vi "configuration UI.vi"() -> ()   [LabVIEW 2013, in "file io module editor node.lvclass"]
uses:
  file io module editor node.lvclass
  <vilib>/NI/DCAF UI Toolkit/Controls/Remove.ctl
  <vilib>/NI/DCAF UI Toolkit/Controls/Add.ctl
  <vilib>/NI/Configuration Framework/Node/NodeRef.ctl
  <vilib>/NI/Configuration Framework/Node/NISE_CEF_Node.lvclass
  <vilib>/NI/AMC/Message Queue.ctl
  <vilib>/NI/AMC/Message.ctl
  <vilib>/NI/Tools/Keyed Array/KeyedArray.ctl
  <vilib>/NI/Configuration Framework/Node/UserEventRef.ctl
  <vilib>/NI/Configuration Framework/Controls/EventCluster.ctl
  <vilib>/NI/Configuration Framework/Node/StopEvent.ctl
  <vilib>/NI/Configuration Framework/Node/RefreshUIEvent.ctl
  <vilib>/NI/Configuration Framework/Node/CacheState.ctl
  <vilib>/NI/Configuration Framework/Node/NodeChangeEvent.ctl
  <vilib>/NI/Tag Bus/tag/Data Type.ctl
  <vilib>/NI/Tag Bus Data Framework/control module/editor node/channel action event.ctl
  <vilib>/NI/Tag Bus Data Framework/control module/editor node/dialog output action.ctl
  <vilib>/NI/Tag Bus Module Framework/channel/TBM channel.lvclass
  <vilib>/NI/Tag Bus/tag/tag descriptor.lvclass
  access.ctl
  <vilib>/NI/DCAF Table API/Table Manager/object ref.ctl
  <vilib>/NI/Tag Bus Data Framework/Configuration Editor/Classes/Engine Parent/Engine Parent Editor Node.lvclass
  <vilib>/NI/Tag Bus Data Framework/Configuration Editor/Classes/Module editor node/module editor node.lvclass
  <vilib>/NI/DCAF Table API/Table Manager/references.ctl
  <vilib>/NI/DCAF Table API/Listbox/Multi Column Listbox.lvclass
  <vilib>/Utility/miscctls.llb/LVPositionTypeDef.ctl
  <vilib>/NI/DCAF Table API/Listbox/Multi Column Listbox.lvclass/Multi Column Listbox.ctl
  <vilib>/NI/DCAF Table API/Table Manager/Table Manager.lvclass/Table Manager.ctl
  <vilib>/NI/DCAF Table API/Listbox/Write Listbox.vi
  <vilib>/NI/DCAF Table API/Table Manager/Write Top VI.vi
  <vilib>/NI/Tag Bus Data Framework/control module/editor node/control module editor.lvclass
  <vilib>/NI/DCAF Table API/Table Manager/Table Manager.lvclass
  <vilib>/NI/Tools/Keyed Array/Tools_KeyedArray.lvlib
  <vilib>/NI/AMC/AMC.lvlib
  <vilib>/NI/Configuration Framework/NISE_CEF_TreeControl.lvlib
  <vilib>/NI/DCAF UI Toolkit/Controls/DCAF UI Elements.lvlib
panel:
  in  "data type":T1
  in  "access":T2
  in  "Top Level Tab Control":enum32{"<Main Page>"}(tab)
  in  "tag list box":i32(listbox)=1
  in  "remove tag":T3
  in  "Add tag":T4
  in  "user event out":refnum<user-event>
  in  "node change":T5
  in  "cache state":T6
  in  "refresh UI":T7
  in  "stop event":T8
  in  "user event":T9
  in  "main queue":T10
  in  "node ref":T11
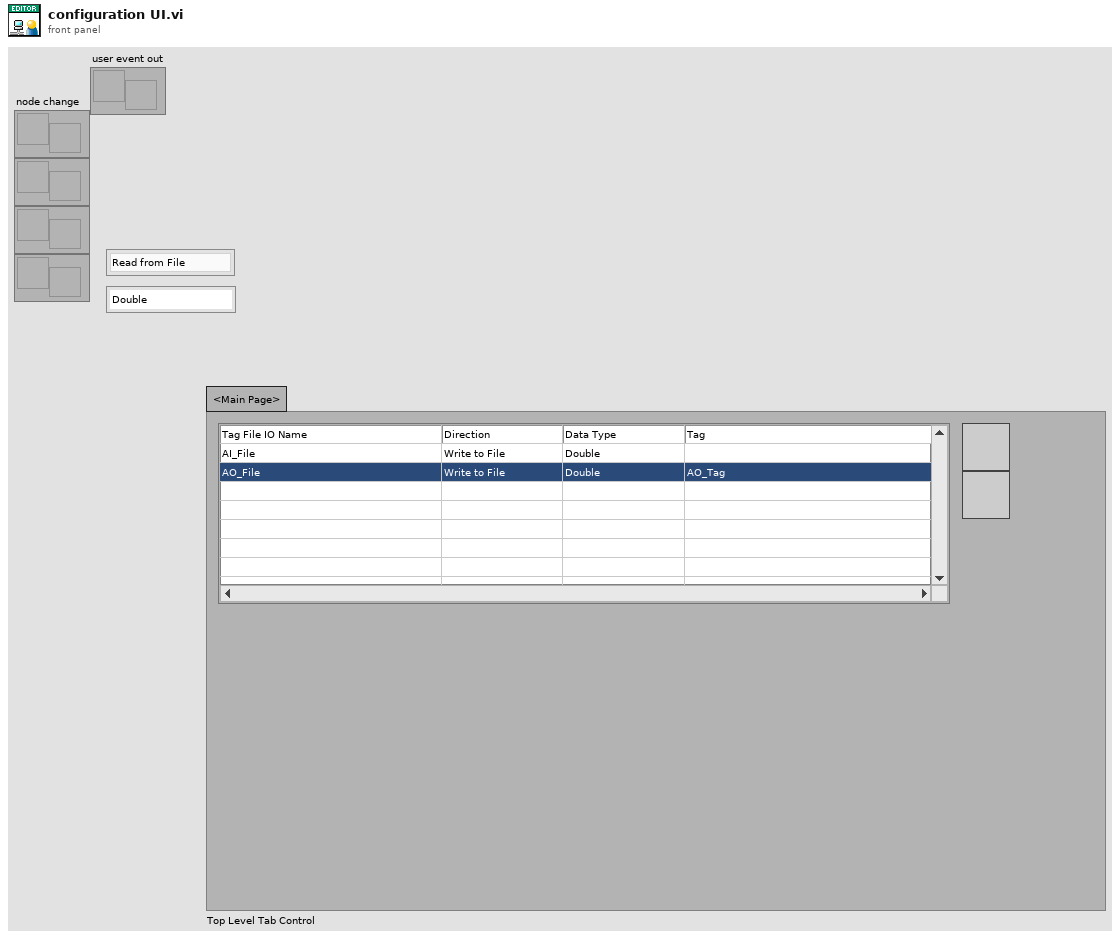
[diagram p1: front panel]
types:
  T1 = typedef "tag bus.lvlib/tag descriptor.lvclass/Data Type.ctl" = enum16{"Double", "Single", "I64", "I32", "I16", "I8", "U64", "U32", "U16", "U8", "Boolean", "String", "Array of Double", "Array of Single", "Array of I64", "Array of I32", "Array of I16", "Array of I8", "Array of U64", "Array of U32", "Array of U16", "Array of U8", "Array of Boolean", "Array of String"}
  T2 = typedef "file io module editor node.lvclass/access.ctl" = enum16{"Read from File", "Write to File"}
  T3 = typedef "DCAF UI Elements.lvlib/Remove.ctl" = bool
  T4 = typedef "DCAF UI Elements.lvlib/Add.ctl" = bool
  T5 = typedef "NISE_CEF_Node.lvclass/NodeChangeEvent.ctl" = refnum<user-event>
  T6 = typedef "NISE_CEF_Node.lvclass/CacheState.ctl" = refnum<user-event>
  T7 = typedef "NISE_CEF_Node.lvclass/RefreshUIEvent.ctl" = refnum<user-event>
  T8 = typedef "NISE_CEF_Node.lvclass/StopEvent.ctl" = refnum<user-event>
  T9 = typedef "NISE_CEF_Node.lvclass/UserEventRef.ctl" = refnum<user-event>
  T10 = typedef "AMC.lvlib/Message Queue.ctl" = refnum<queue>
  T11 = typedef "NISE_CEF_Node.lvclass/NodeRef.ctl" = refnum<data-value>
  T12 = typedef "LVPositionTypeDef.ctl" = cluster{"Left":i32, "Top":i32}
  T13 = typedef "Table Manager.lvlib/Table Manager.lvclass/references.ctl" = cluster{"stop event":T8, "refresh UI":T7, "cache state":T6, "node change":T5, "user event out":refnum<user-event>, "main queue":T10, "user event":T9}
  T14 = typedef "Table Manager.lvlib/Table Manager.lvclass/object ref.ctl" = cluster{"engine":refnum<data-value>, "Node Ref":refnum<data-value>}
  T15 = typedef "Table Manager.lvlib/Column.lvclass/Column Descriptor.ctl" = cluster{"name":string, "caption":string, "Column Type":T16, "Params":string, "AutoSizeMode":i32, "FillWeight":sgl, "MinWidth":u32, "tooltip":string, "Enum Reference":refnum<vi>, "Channel suffix":string, "Read Only":bool, "Call Back VI":T17, "DT Dependency":i32, "name dependency":i32, "data type":T1}
  T16 = typedef "Table Manager.lvlib/Column.lvclass/Column Type.ctl" = enum16{"String", "Mapping", "Channel Name", "Tag", "Enum", "Data Type", "Numeric"}
  T17 = typedef "Table Manager.lvlib/Table Manager.lvclass/Call Back Ref Type Def.ctl" = refnum<vi>
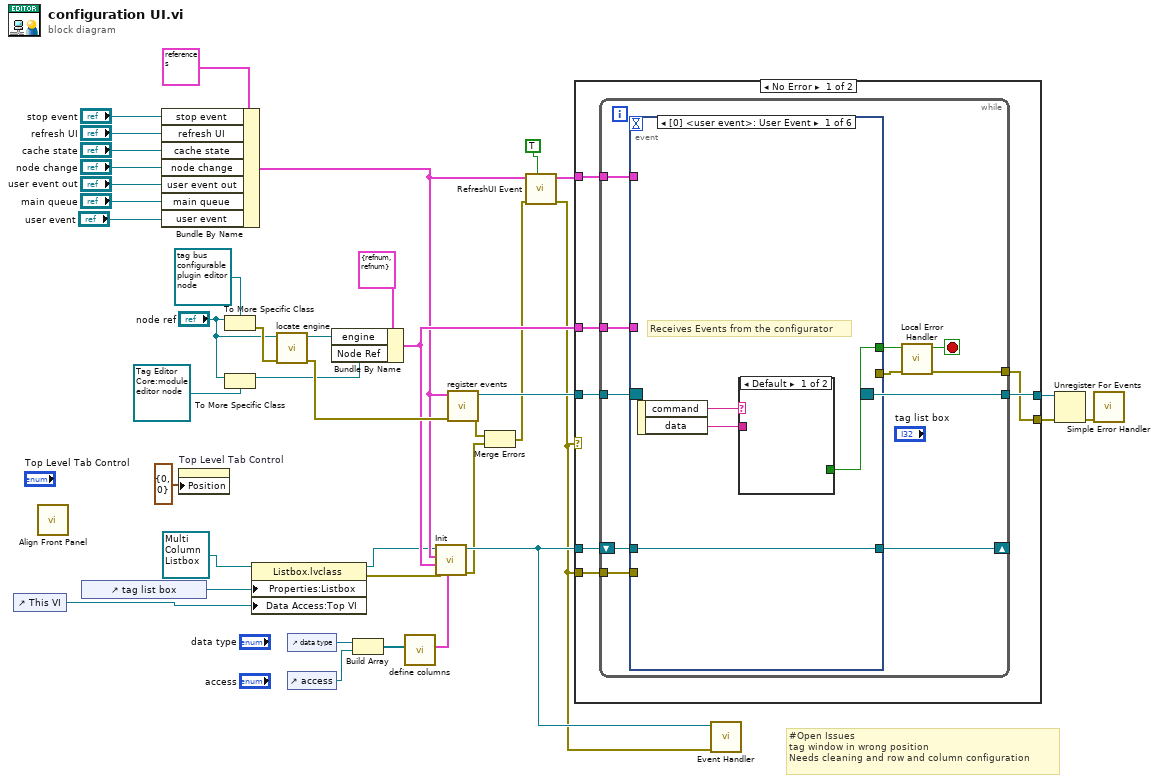
[diagram p0: block diagram]
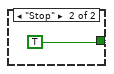
[diagram p2: hidden frame]
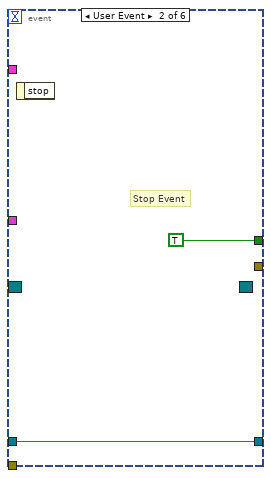
[diagram p3: hidden frame]
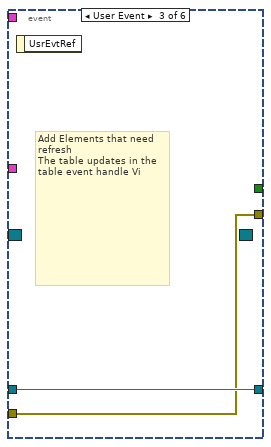
[diagram p4: hidden frame]
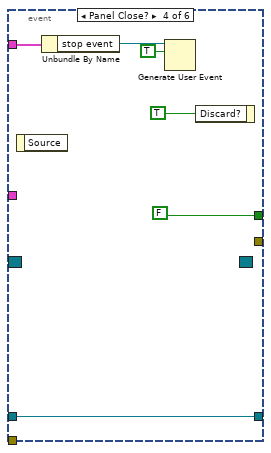
[diagram p5: hidden frame]
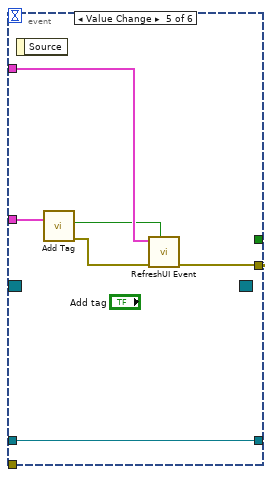
[diagram p6: hidden frame]
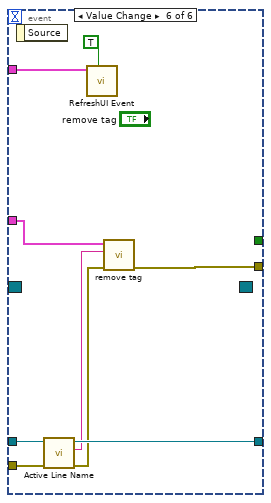
[diagram p7: hidden frame]
diagram:
  # "#Open Issues \ntag window in wrong position\nNeeds cleaning and row and column configuration"
  n1 = control-ref of="This VI"() -> (w15:refnum<vi>)
  n2 = call <vilib>:"Align Front Panel.vi"() -> ()  [unwired: 10 in, 2 out]
  n3 = control-ref of="tag list box"() -> (w16:refnum<vi>)
  n4 = Bundle By Name(cluster=T13 {"stop event"=refnum, "refresh UI"=refnum, "cache state"=refnum, "node change"=refnum, "user event out"=refnum, "main queue"=refnum, "user event"=refnum} ("References"), "stop event"="stop event", "refresh UI"="refresh UI", "cache state"="cache state", "node change"="node change", "user event out"="user event out", "main queue"="main queue", "user event"="user event") -> (w13:T13)
  n5 = property on="Top Level Tab Control" class="TabCtl (strict)"("Position"=T12 {"Left"=0, "Top"=0}) -> ()  [unwired: 2 in, 2 out]
  n6 = To More Specific Class(target class=refnum<data-value> refnum ("data value reference"), reference="node ref") -> (error out=w24:errorcluster)  [unwired: 1 in, 1 out]
  n7 = To More Specific Class(target class=refnum<data-value> refnum ("data value reference"), reference="node ref") -> (specific class reference=w6:refnum<data-value>)  [unwired: 1 in, 1 out]
  n8 = property class="Listbox.lvclass"(reference=refnum<class "Multi Column Listbox.lvclass"> refnum ("Table Manager.lvlib:Multi Column Listbox.lvclass"), "Properties:Listbox"=w16, "Data Access:Top VI"=w15) -> (reference out=w5:refnum<class "Multi Column Listbox.lvclass">, error out=w20:errorcluster)  [unwired: 1 in]
  n9 = call <vilib>:"locate engine.vi"("error in"=w24, "component"="node ref") -> ("error out"=w21:errorcluster, "engine"=w23:refnum<data-value>)  [unwired: 8 in]
  n10 = control-ref of="data type"() -> (w2:refnum<vi>)
  n11 = control-ref of="access"() -> (w4:refnum<vi>)
  n12 = Bundle By Name(cluster=T14 {"engine"=refnum, "Node Ref"=refnum} ("references"), "engine"=w23, "Node Ref"=w6) -> (w14:T14)
  n13 = Build Array(w2, w4) -> (w1:refnum<vi>[])
  n14 = call "define columns.vi"("enum references"=w1) -> ("Column Definition"=w19:T15[])  [unwired: 10 in]
  n15 = call-dynamic "Init.vi"("Column Definitions"=w19, "error in (no error)"=w20, "object refs"=w14, "References in"=w13, "Multi Column Listbox in"=w5) -> ("error out"=w12:errorcluster, "Multi Column Listbox out"=w34:refnum<class "Multi Column Listbox.lvclass">)  [unwired: 4 in, 1 out]
  n16 = call "register events.vi"("error in (no error)"=w21, "References"=w13) -> ("error out"=w11:errorcluster, "Event Registration Refnum"=w36:refnum<event-registration>)  [unwired: 8 in]
  n17 = Merge Errors(w11, w12) -> (w10:errorcluster)
  n18 = call "RefreshUI Event.vi"("Refresh?"=TRUE, "error in"=w10, "References in"=w13) -> ("error out"=w9:errorcluster, "References out"=w35:T13)  [unwired: 7 in]
  n19 = case shown="No Error" w9 {
    selector: w9 -> [_ w89]
    tunnel: w36 -> [w46 w88]
    tunnel: [w45 w88] -> w39
    tunnel: [w44 w89] -> w38
    tunnel: w35 -> [w43 _]
    tunnel: w14 -> [w42 _]
    tunnel: w34 -> [w41 _]
    tunnel: w9 -> [w40 _]
    frame No Error {
      n20 = while {
        tunnel: w46 -> [w57]
        tunnel: [w56] -> w45
        tunnel: [w53] -> w44
        tunnel: w43 -> [w51]
        tunnel: w42 -> [w50]
        shift-right: [w48] -> _
        shift-left: w41 -> [w49]
        tunnel: w40 -> [w47]
        stop <- w55 stop-if-true
        n21 = event shown="[0] <user event>: User Event" {
          selector: w57 -> [_ _ _ _ _ _]
          dyn-events: [_ _ _ _ _ _] -> w56
          timeout: _ -> [_ _ _ _ _ _]
          tunnel: [w61 TRUE _ FALSE _ _] -> w54
          tunnel: [_ _ w65 _ w74 w87] -> w52
          tunnel: w51 -> [_ _ _ w68 w77 w85]
          tunnel: w50 -> [_ _ _ _ w73 w84]
          tunnel: w49 -> [w58 w63 w66 w67 w78 w83]
          tunnel: [w58 w63 w66 w67 w78 w81] -> w48
          tunnel: w47 -> [_ _ w65 _ _ w82]
          event User Event {
            # "Receives Events from the configurator"
            n22 = event-data() -> ("command"=w60:string, "data"=w59:string)  [unwired: 1 in]
            n23 = case shown="Default" w60 {
              tunnel: [_ TRUE] -> w61
              tunnel: w59 -> [_ _]
              frame Default {
              }
              frame "Stop" {
              }
            }
          }
          event User Event {
            # "Stop Event"
            n24 = event-data() -> ()  [unwired: 1 in, 1 out]
          }
          event User Event {
            # "Add Elements that need refresh \nThe table updates in the table event handle Vi"
            n25 = event-data() -> ()  [unwired: 1 in, 1 out]
          }
          event Panel Close? {
            n26 = event-data() -> ()  [unwired: 1 in, 1 out]
            n27 = Unbundle By Name(w68) -> ("stop event"=w69:T8)
            n28 = Generate User Event(user event=w69, event data cluster=TRUE ("event data")) -> ()  [unwired: 2 in, 2 out]
            n29 = event-data("Discard?"=TRUE) -> ()  [unwired: 1 in, 1 out]
          }
          event Value Change {
            n30 = event-data() -> ()  [unwired: 1 in, 1 out]
            n31 = call "Add Tag.vi"("references"=w73) -> ("error out"=w75:errorcluster, "newtag?"=w76:bool)  [unwired: 9 in]
            n32 = call "RefreshUI Event.vi"("Refresh?"=w76, "error in"=w75, "References in"=w77) -> ("error out"=w74:errorcluster)  [unwired: 7 in, 1 out]
          }
          event Value Change {
            n33 = event-data() -> ()  [unwired: 1 in, 1 out]
            n34 = call-dynamic "Active Line Name.vi"("error in"=w82, "Multi Column Listbox in"=w83) -> ("error out"=w79:errorcluster, "Active Line Name"=w80:string, "Multi Column Listbox out"=w81:refnum<class "Multi Column Listbox.lvclass">)  [unwired: 7 in]
            n35 = call "RefreshUI Event.vi"("Refresh?"=TRUE, "References in"=w85) -> ()  [unwired: 8 in, 2 out]
            n36 = call "remove tag.vi"("error in"=w79, "tag"=w80, "object ref in"=w84) -> ("error out"=w87:errorcluster)  [unwired: 8 in]
          }
        }
        n37 = call "Local Error Handler.vi"("error in"=w52, "stop in"=w54) -> ("error out"=w53:errorcluster, "stop out"=w55:bool)  [unwired: 8 in]
      }
    }
    frame Error {
    }
  }
  n38 = call-dynamic "Event Handler.vi"("error in"=w9, "Listbox in"=w34) -> ()  [unwired: 8 in, 2 out]
  n39 = Unregister For Events(event registration refnum=w39, error in=w38) -> (error out=w37:errorcluster)
  n40 = call <vilib>:"Simple Error Handler.vi"("error in (no error)"=w37) -> ()  [unwired: 4 in, 5 out]
